vi "Configure LXI.vi"(8 "error in (no error)":errorcluster, 9 "Enable Multicast DNS Service (T: Enable)":bool=TRUE, 10 "LXI Status (0: No Fault)":i32(ring) items=["No Fault", "Identify"], 11 "VISA resource name":refnum<visa-resource-name>) -> (0 "error out":errorcluster, 3 "VISA resource name out":refnum<visa-resource-name>)   [LabVIEW 2020, in "Keysight E36300 Series.lvlib"]
doc: "Configures the LXI attribute.\n\n<b>Note: </b>\nThis VI is only available on the E36312A and E36313A models."
uses:
  Keysight E36300 Series.lvlib
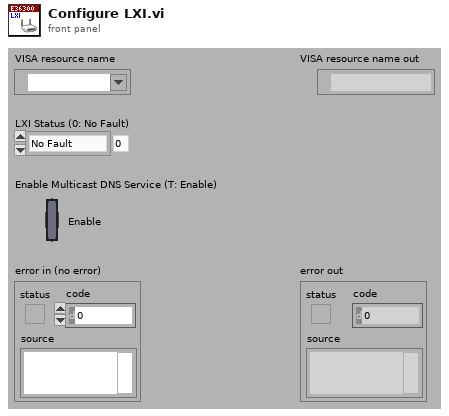
[diagram p1: front panel]
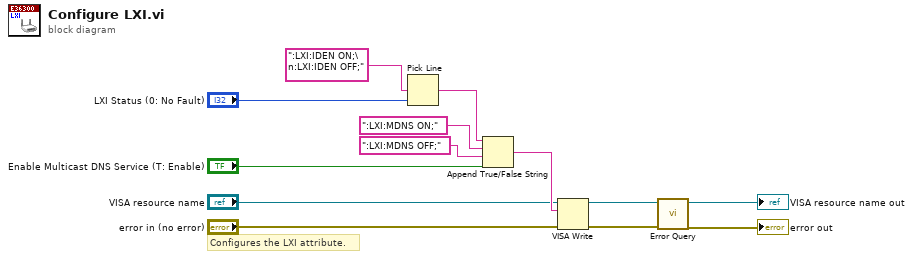
[diagram p0: block diagram]
diagram:
  # "Configures the LXI attribute."
  n1 = Pick Line(multi-line string=":LXI:IDEN ON;\n:LXI:IDEN OFF;", line index="LXI Status (0: No Fault)") -> (output string=w11:string)  [unwired: 1 in]
  n2 = Append True/False String(1:"Enable Multicast DNS Service (T: Enable)", 2:":LXI:MDNS OFF;", 3:":LXI:MDNS ON;", 4:w11) -> (0:w7:string)
  n3 = VISA Write(VISA resource name="VISA resource name", write buffer=w7, error in (no error)="error in (no error)") -> (VISA resource name out=w4:refnum<visa-resource-name>, error out=w3:errorcluster)  [unwired: 1 out]
  n4 = call "Error Query.vi"("error in (no error)"=w3, "VISA resource name"=w4) -> ("error out"=→"error out":errorcluster, "VISA resource name out"=→"VISA resource name out":refnum<visa-resource-name>)  [unwired: 6 in, 2 out]
